vi "lab_3_partie_1 - Copie.vi"() -> ()   [LabVIEW 2020]
uses:
  <instrlib>/Agilent 34401/Public/Data/Read (Single Point).vi
  <instrlib>/Agilent E363X Series/Agilent E363X Series.lvlib
  <instrlib>/Agilent 34401/Agilent 34401.lvlib
panel:
  out "XY Graph":cluster{"Y":dbl[], "Y":dbl[]}[](graph) caption="Graphe XY"
  in  "Tension maximale":dbl(slide) scale=0.0..6.0
  out "Courant":dbl
  in  "Incrément \ntension":sgl step=0.05
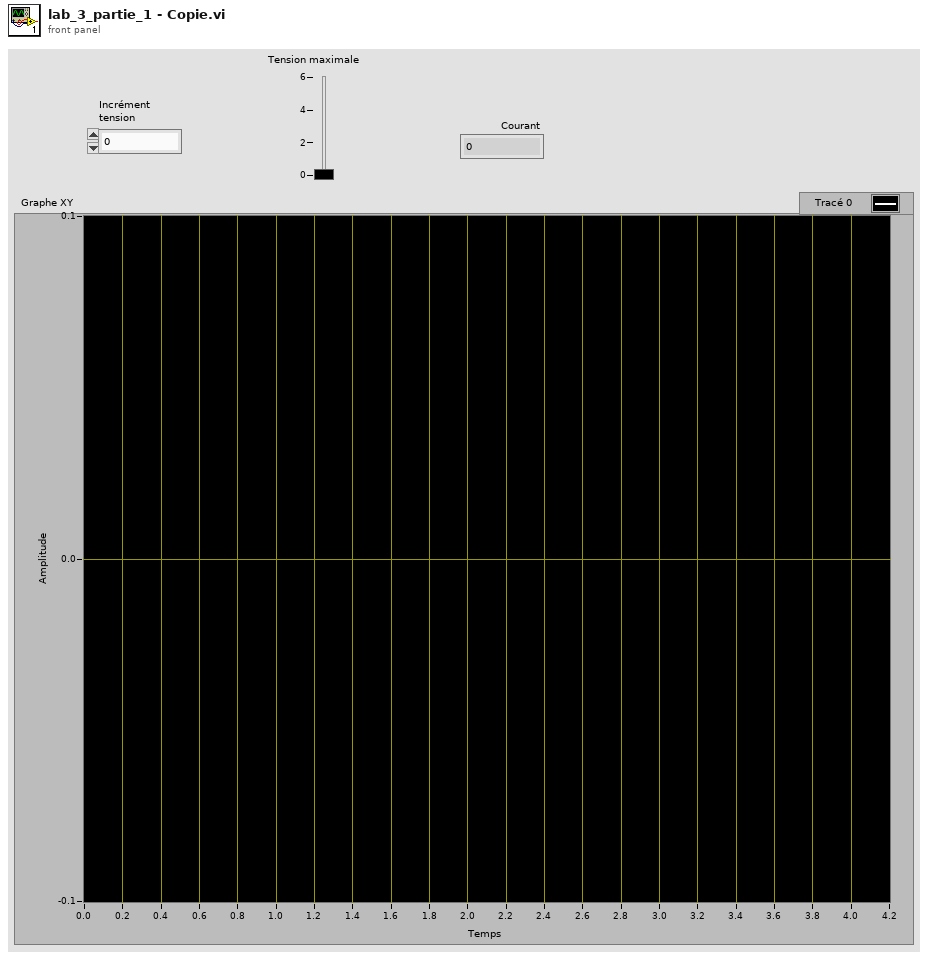
[diagram p1: front panel]
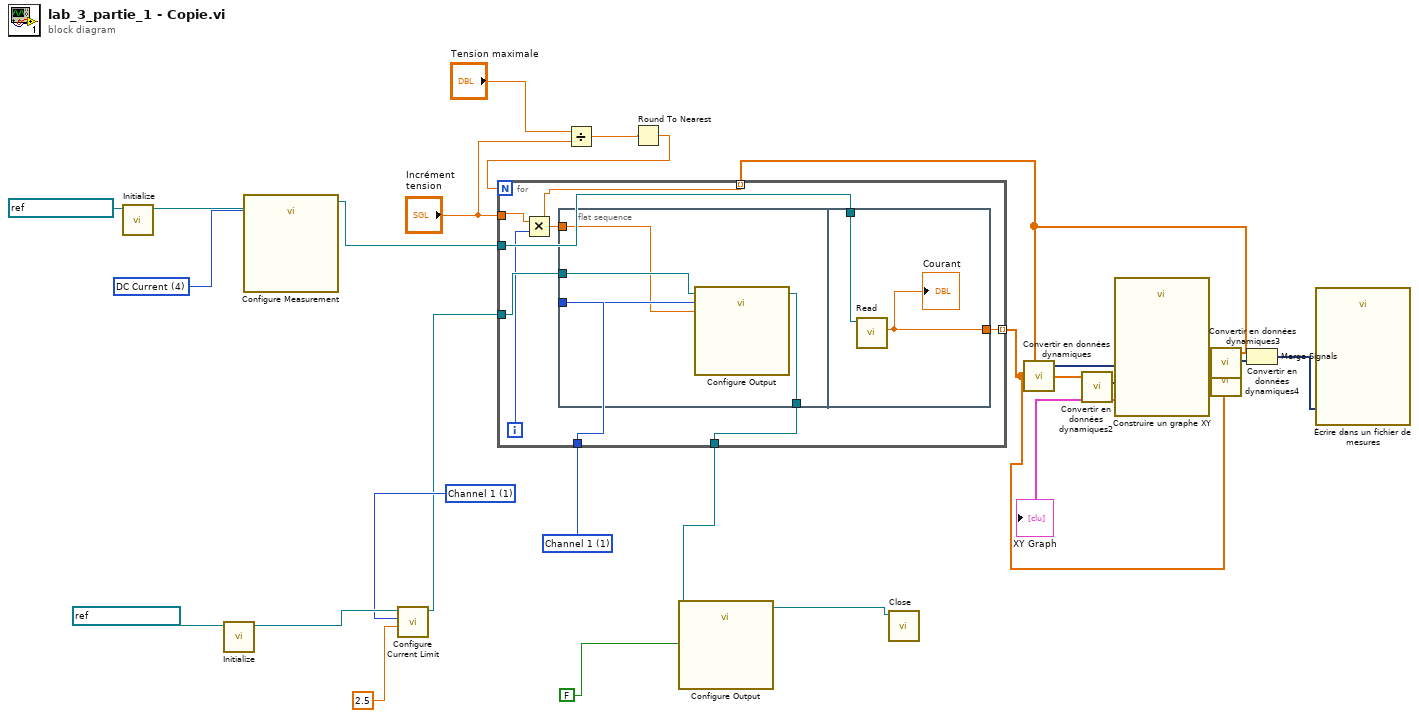
[diagram p0: block diagram]
diagram:
  w19 = u16 4 items=["DC Voltage", "AC Voltage", "2 - Wire Resistance", "4 - Wire Resistance", "DC Current", "AC Current", "Frequency", "Period", "Continuity", "Diode Checking", "VDC:VDC Ratio", "Temperature", "Capacitance"] ("Function (0: DC Voltage)")
  w17 = 1 items=["Channel 1"=1, "Channel 2"=2, "Channel 3"=3] ("Channel (1: Channel 1)")
  w22 = 1 items=["Channel 1"=1, "Channel 2"=2, "Channel 3"=3] ("Channel (1: Channel 1)")
  n1 = call <instrlib>:"Initialize.vi"("VISA resource name"=refnum<visa-resource-name> "GPIB0::22::INSTR") -> ("VISA resource name out"=w20:refnum<visa-resource-name>)  [unwired: 9 in, 1 out]
  n2 = call <instrlib>:"Initialize.vi"("VISA resource name"=refnum<visa-resource-name> "GPIB0::5::INSTR") -> ("VISA resource name out"=w24:refnum<visa-resource-name>)  [unwired: 9 in, 1 out]
  n3 = call <instrlib>:"Configure Measurement.vi"("Function (0: DC Voltage)"=w19, "VISA resource name"=w20) -> ("VISA resource name out"=w14:refnum<visa-resource-name>)  [unwired: 8 in, 1 out]
  n4 = call <instrlib>:"Configure Current Limit.vi"("Current Limit (0.0 A)"=2.5, "Channel (1: Channel 1)"=w22, "VISA resource name"=w24) -> ("VISA resource name out"=w16:refnum<visa-resource-name>)  [unwired: 7 in, 1 out]
  n5 = Divide(x="Tension maximale", y="Incrément \ntension") -> (x/y=w11:dbl)
  n6 = Round To Nearest(number=w11) -> (nearest integer value=w10:dbl)
  n7 = for {
    N: w10 -> [_]
    tunnel: w17 -> [w33]
    tunnel: w16 -> [w32]
    tunnel: [w31] -> w15
    tunnel: w14 -> [w30]
    tunnel: "Incrément \ntension" -> [w29]
    tunnel: [w27] -> w5 mode=indexing
    tunnel: [w26] -> w3 mode=indexing
    i -> [w28]
    n8 = Multiply(x=w29, y=w28) -> (x*y=w27:sgl)
    n9 = flat-sequence {
      tunnel: w33 -> [w37]
      tunnel: w32 -> [w36]
      tunnel: [w35] -> w31
      tunnel: w27 -> [w34]
      tunnel: w30 -> [w39]
      tunnel: [w38] -> w26
      frame #0 {
        n10 = call <instrlib>:"Configure Output.vi"("Voltage Level (0.0 V)"=w34, "Channel (1: Channel 1)"=w37, "VISA resource name"=w36) -> ("VISA resource name out"=w35:refnum<visa-resource-name>)  [unwired: 7 in, 1 out]
      }
      frame #1 {
        n11 = call-poly <instrlib>:"Read.vi"("VISA resource name"=w39) -> ("Measurement"=w38:dbl)  [unwired: 8 in, 2 out]
        "Courant" <- w38
      }
    }
  }
  n12 = call <instrlib>:"Configure Output.vi"("Enable Output (T: Enable)"=FALSE, "VISA resource name"=w15) -> ("VISA resource name out"=w18:refnum<visa-resource-name>)  [unwired: 8 in, 1 out]
  n13 = call <instrlib>:"Close.vi"("VISA resource name"=w18) -> ()  [unwired: 10 in, 1 out]
  n14 = call "Convertir en données dynamiques"("Array"=w5) -> ("Dynamic Data Type"=w8:dynamicdata)  [unwired: 3 in]
  n15 = call "Convertir en données dynamiques2"("Array"=w3) -> ("Dynamic Data Type"=w7:dynamicdata)  [unwired: 3 in]
  n16 = call "Construire un graphe XY"("Y Input"=w7, "X Input"=w8) -> ("XY Graph"=→"XY Graph":cluster{"X":dbl[], "Y":dbl[]}[])  [unwired: 8 in, 1 out]
  n17 = call "Convertir en données dynamiques3"("Array"=w5) -> ("Dynamic Data Type"=w4:dynamicdata)  [unwired: 3 in]
  n18 = call "Convertir en données dynamiques4"("Array"=w3) -> ("Dynamic Data Type"=w2:dynamicdata)  [unwired: 3 in]
  n19 = Merge Signals(w4, w2) -> (w6:dynamicdata)
  n20 = call "Écrire dans un fichier de mesures"("Signals"=w6) -> ()  [unwired: 16 in, 3 out]
